vi "control_zone.vi"(1 "duty cycle in":dbl, 4 "Channel":i32, 6 "total cycle time":dbl=10.0, 7 "Last State":bool, 8 "error in":errorcluster, 9 "Seq Start Time":dbl, 10 "Now Time":dbl, 11 "Handle In":i32) -> (0 "error out":errorcluster, 3 "Handle Out":i32, 5 "state out":bool)   [LabVIEW 2020]
panel:
  out "Zone 1 Duty Cycle":dbl(knob) scale=0.0..100.0
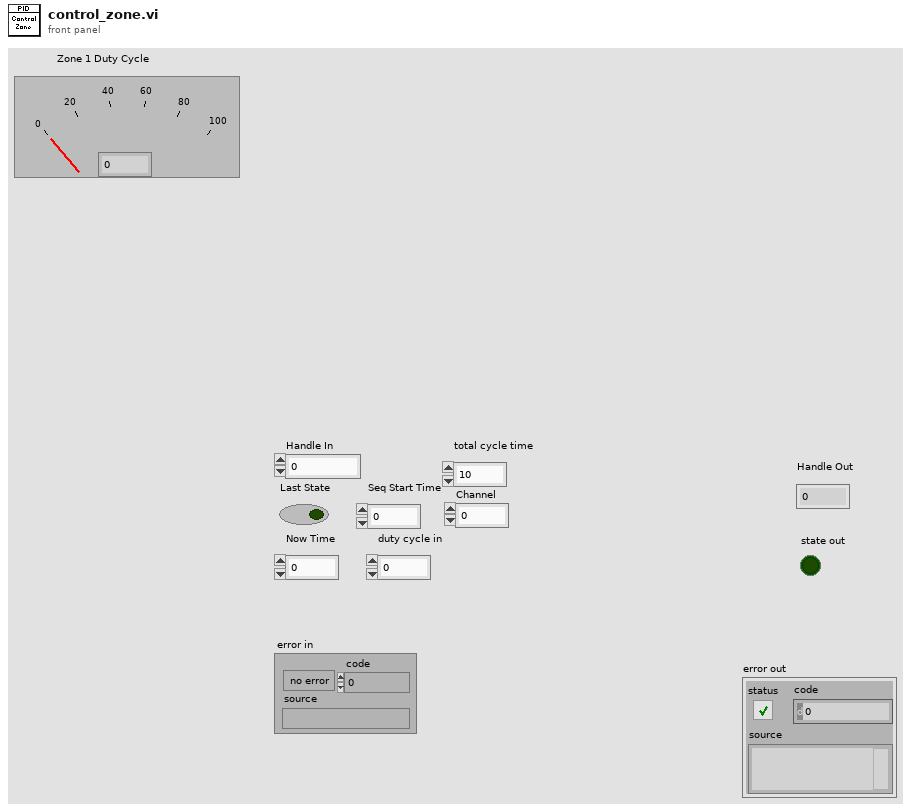
[diagram p1: front panel]
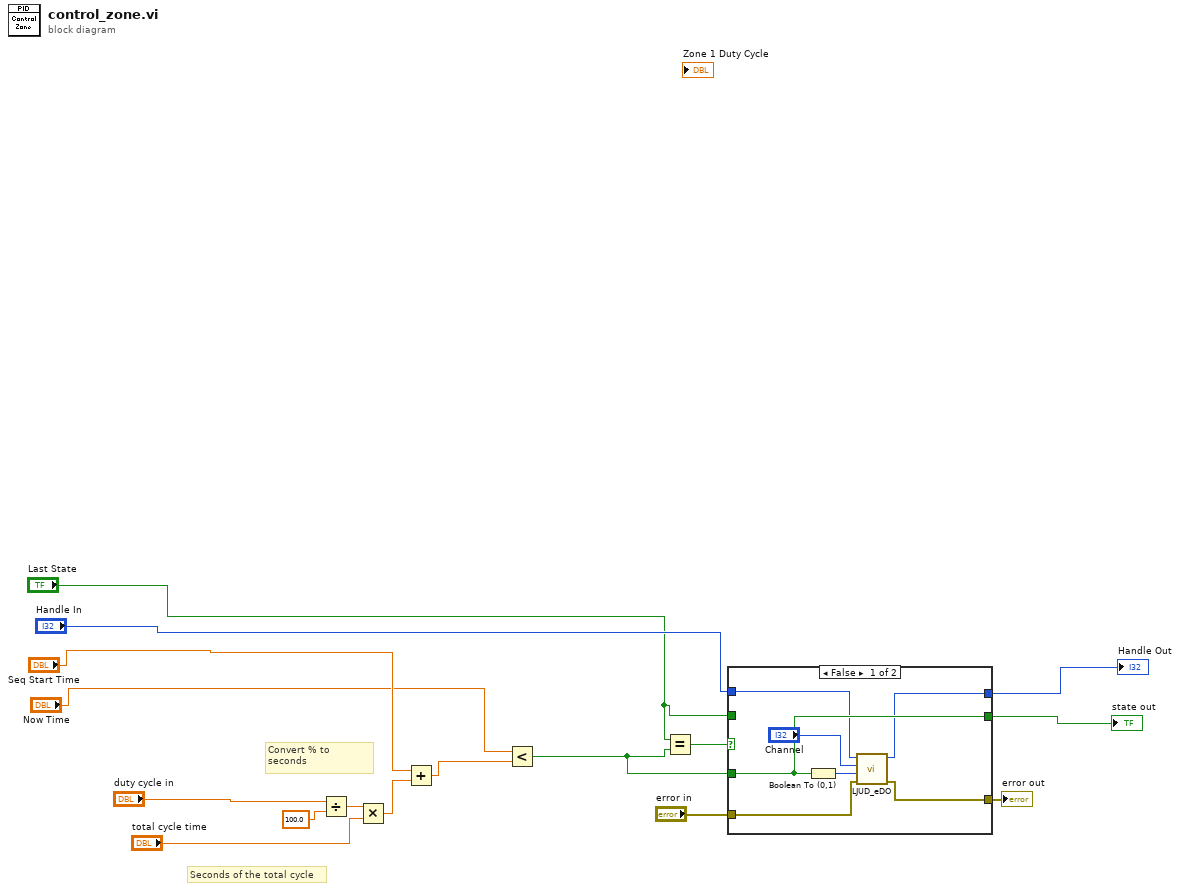
[diagram p0: block diagram]
diagram:
  # "Convert % to seconds"
  # "Seconds of the total cycle"
  n1 = Divide(x="duty cycle in", y=100.0) -> (x/y=w15:dbl)
  n2 = Multiply(x=w15, y="total cycle time") -> (x*y=w14:dbl)
  n3 = Add(x="Seq Start Time", y=w14) -> (x+y=w13:dbl)
  n4 = Less?(x="Now Time", y=w13) -> (x < y?=w11:bool)
  n5 = Equal?(x="Last State", y=w11) -> (x = y?=w12:bool)
  n6 = case shown="False" w12 {
    tunnel: [w22 w26] -> w2
    tunnel: "Last State" -> [_ w26]
    tunnel: w11 -> [w22 _]
    tunnel: "Handle In" -> [w21 w25]
    tunnel: [w20 w25] -> w9
    tunnel: [w19 w24] -> w3
    tunnel: "error in" -> [w18 w24]
    frame False {
      n7 = Boolean To (0,1)(Boolean=w22) -> (0, 1=w23:i16)
      n8 = call "LJUD_eDO.vi"("error in"=w18, "State"=w23, "Channel"="Channel", "Handle In"=w21) -> ("error out"=w19:errorcluster, "Handle Out"=w20:i32)  [unwired: 6 in]
    }
    frame True {
      # "Already in correct state"
    }
  }
  "Handle Out" <- w9
  "error out" <- w3
  "state out" <- w2
